vi "Write File.vi"(8 "error in":errorcluster, 11 "tCRD in":refnum<class "Open Path CRD.lvclass">) -> (0 "error out":errorcluster, 3 "tCRD out":refnum<class "Open Path CRD.lvclass">)   [LabVIEW 2015, in "Open Path CRD.lvclass"]
uses:
  Open Path CRD.lvclass
  Reusable/File IO/Class/File Observer.lvclass
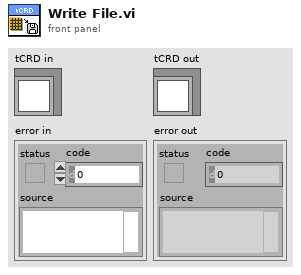
[diagram p1: front panel]
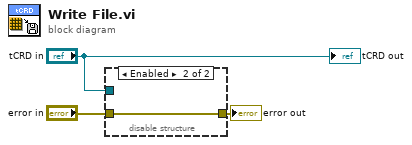
[diagram p0: block diagram]
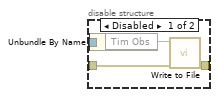
[diagram p2: hidden frame]
diagram:
  n1 = disable-structure shown="Enabled" {
    disable-tunnel: "error in" -> [w6 w8]
    disable-tunnel: [w5 w8] -> w2
    disable-tunnel: "tCRD in" -> [w4 _]
    frame Disabled {
      n2 = Unbundle By Name(w4) -> ("Tim Obs"=w7:refnum<class "Tim File Observer.lvclass">)
      n3 = call "Write to File.vi"("error in"=w6, "File Obs in"=w7) -> ("error out"=w5:errorcluster)  [unwired: 8 in, 1 out]
    }
    frame Enabled {
    }
  }
  "error out" <- w2
  "tCRD out" <- "tCRD in"
